vi "SwerveSetPointEditing.vi"(10 "pv":dbl, 11 "theta":dbl) -> (2 "sp":dbl, 3 "Boolean":bool)   [LabVIEW 2017]
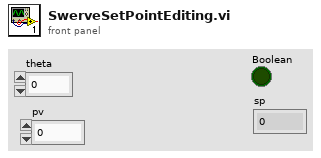
[diagram p1: front panel]
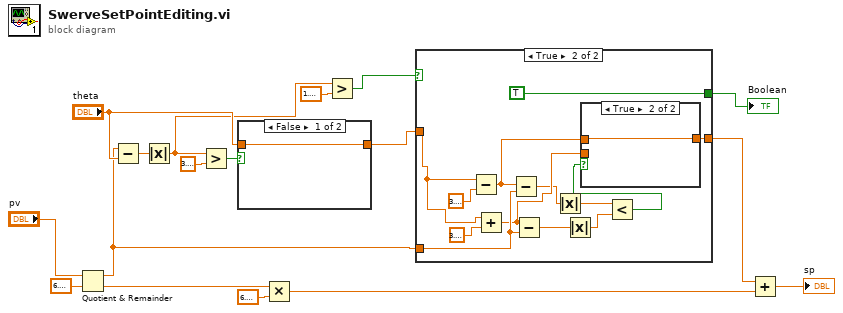
[diagram p0: block diagram]
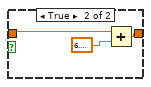
[diagram p2: hidden frame]
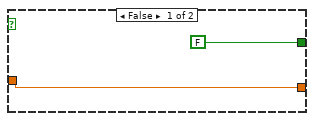
[diagram p3: hidden frame]
diagram:
  n1 = Quotient & Remainder(x="pv", y=6.283185307179586) -> (x-y*floor(x/y)=w1:dbl, floor(x/y)=w4:dbl)
  n2 = Subtract(x=w1, y="theta") -> (x-y=w16:dbl)
  n3 = Absolute Value(x=w16) -> (abs(x)=w3:dbl)
  n4 = Greater?(x=w3, y=3.141592653589793) -> (0:w11:bool)
  n5 = case shown="False" w11 {
    tunnel: "theta" -> [w18 w20]
    tunnel: [w18 w19] -> w9
    frame False {
    }
    frame True {
      n6 = Add(x=w20, y=6.283185307179586) -> (x+y=w19:dbl)
    }
  }
  n7 = Multiply(x=w4, y=6.283185307179586) -> (x*y=w6:dbl)
  n8 = Greater?(x=w3, y=1.5707963267948966) -> (0:w14:bool)
  n9 = case shown="True" w14 {
    tunnel: [w22 w31] -> w7
    tunnel: [FALSE TRUE] -> w15
    tunnel: w9 -> [w22 w34]
    tunnel: w1 -> [_ w33]
    frame False {
    }
    frame True {
      n10 = Subtract(x=w34, y=3.141592653589793) -> (x-y=w30:dbl)
      n11 = Add(x=w34, y=3.141592653589793) -> (x+y=w29:dbl)
      n12 = Subtract(x=w30, y=w33) -> (x-y=w28:dbl)
      n13 = Subtract(x=w29, y=w33) -> (x-y=w26:dbl)
      n14 = Absolute Value(x=w28) -> (abs(x)=w27:dbl)
      n15 = Absolute Value(x=w26) -> (abs(x)=w25:dbl)
      n16 = Less?(x=w27, y=w25) -> (x < y?=w32:bool)
      n17 = case shown="True" w32 {
        tunnel: [w37 w38] -> w31
        tunnel: w30 -> [_ w38]
        tunnel: w29 -> [w37 _]
        frame False {
        }
        frame True {
        }
      }
    }
  }
  "Boolean" <- w15
  n18 = Add(x=w7, y=w6) -> (x+y=→"sp":dbl)
